vi "SID calc filter freq.vi"(11 "x value":dbl format="%0.2f") -> (3 "interpolation value":dbl format="%0.2f")   [LabVIEW 2018]
uses:
  <vilib>/gmath/NI_Gmath.lvlib
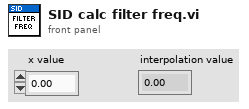
[diagram p1: front panel]
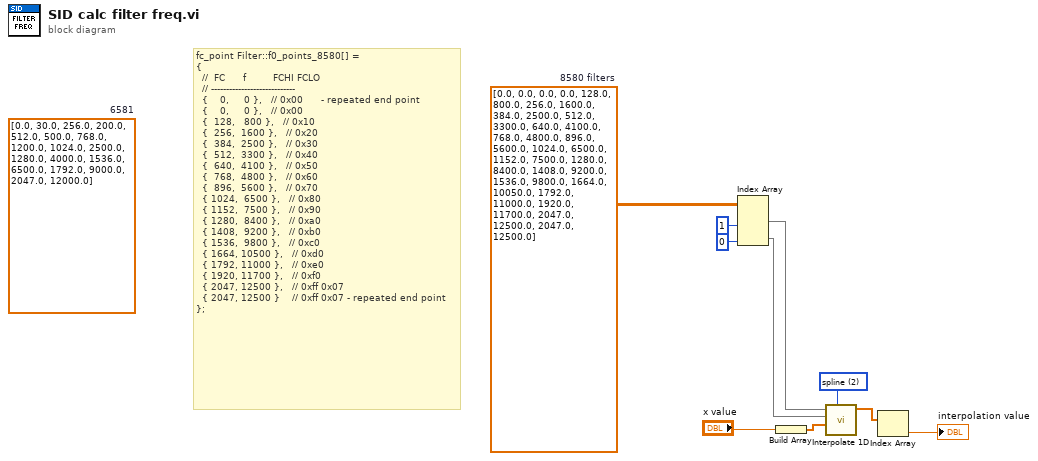
[diagram p0: block diagram]
diagram:
  w3 = 2 items=["nearest", "linear", "spline", "cubic Hermite", "Lagrange"] ("method")
  (unwired) dbl[][] [[0.0, 30.0], [256.0, 200.0], [512.0, 500.0], [768.0, 1200.0], [1024.0, 2500.0], [1280.0, 4000.0], [1536.0, 6500.0], [1792.0, 9000.0], [2047.0, 12000.0]]  # 6581
  w1 = dbl[][] [[0.0, 0.0], [0.0, 0.0], [128.0, 800.0], [256.0, 1600.0], [384.0, 2500.0], [512.0, 3300.0], [640.0, 4100.0], [768.0, 4800.0], [896.0, 5600.0], [1024.0, 6500.0], [1152.0, 7500.0], [1280.0, 8400.0], [1408.0, 9200.0], [1536.0, 9800.0], [1664.0, 10050.0], [1792.0, 11000.0], [1920.0, 11700.0], [2047.0, 12500.0], [2047.0, 12500.0]]  # 8580 filters
  # "fc_point Filter::f0_points_8580[] =\n{\n  //  FC      f         FCHI FCLO\n  // ----------------------------\n  {    0,     0 },   // 0x00      - repeated end point\n  {    0,     0 },   // 0x00\n  {  128,   800 },   // 0x10\n  {  256,  1600 },   // 0x20\n  {  384,  2500 },   // 0x30\n  {  512,  3300 },   // 0x40\n  {  640,  4100 },   // 0x50\n  {  768,  4800 },   // 0x60\n  {  896,  5600 },   // 0x70\n  { 1024,  6500 },   // 0x80\n  { 1152,  7500 },   // 0x90\n  { 1280,  8400 },   // 0xa0\n  { 1408,  9200 },   // 0xb0\n  { 1536,  9800 },   // 0xc0\n  { 1664, 10500 },   // 0xd0\n  { 1792, 11000 },   // 0xe0\n  { 1920, 11700 },   // 0xf0\n  { 2047, 12500 },   // 0xff 0x07\n  { 2047, 12500 }    // 0xff 0x07 - repeated end point\n};"
  n1 = Index Array(array=w1, index (col) #1=1 ("disabled index (col)"), index (col) #2=0 ("index (col)")) -> (element #1=w8:dbl[], element #2=w7:dbl[])  [unwired: 2 in]
  n2 = Build Array("x value") -> (w5:dbl[])
  n3 = call <vilib>:"Interpolate 1D.vi"("method"=w3, "xi"=w5, "X"=w7, "Y"=w8) -> ("yi"=w4:dbl[])  [unwired: 5 in, 2 out]
  n4 = Index Array(array=w4) -> (element=→"interpolation value":dbl)  [unwired: 1 in]
